vi "Fit VI window to Largest Dec.vi"(4 "error in (no error)":errorcluster, 6 "border spacing (2 px)":i32=2, 7 "VI Ref (calling VI)":refnum<vi>) -> (0 "error out":errorcluster, 3 "dup VI Ref":refnum<vi>)   [LabVIEW 2019]
doc: "This utility will fit (resize and center) a VI (defined by the \"VI Ref\" input) about the largest decoration in that VI. It will add a border defined by border spacing in units of pixels. If there are no decorations found in the VI it is a no-op and will not produce an error. Unfortunately, this VI can not find locked decorations (yet)."
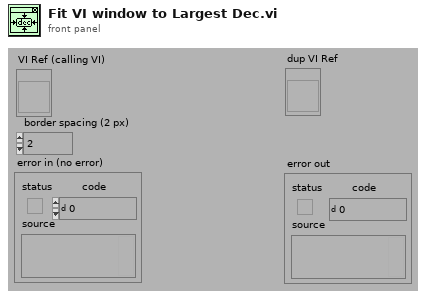
[diagram p1: front panel]
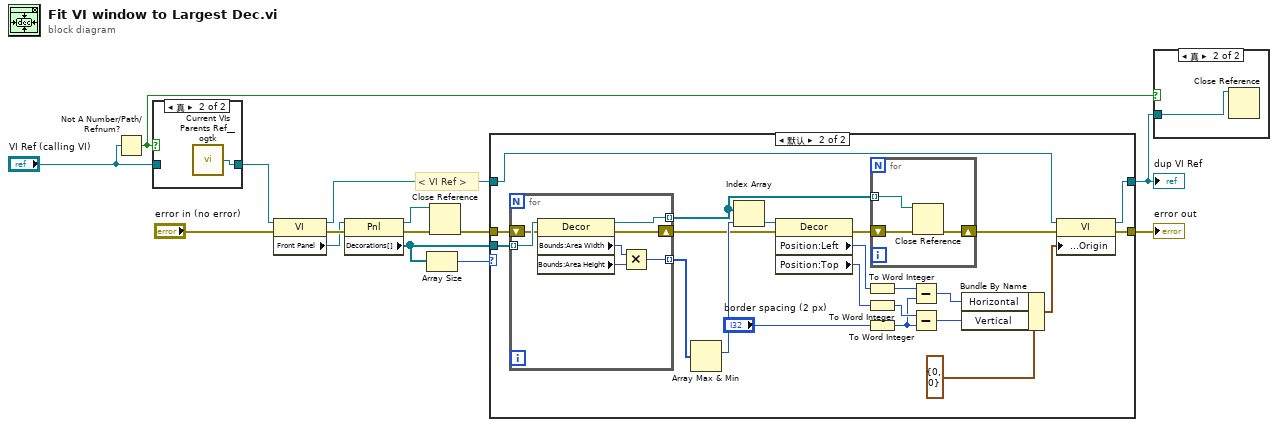
[diagram p0: block diagram]
diagram:
  # "< VI Ref >"
  n1 = Not A Number/Path/Refnum?(number/path/refnum="VI Ref (calling VI)") -> (NaN/Path/Refnum?=w2:bool)
  n2 = case shown="真" w2 {
    tunnel: [w15 w16] -> w3
    tunnel: "VI Ref (calling VI)" -> [w15 _]
    frame False {
    }
    frame True {
      n3 = call <userlib>:"Current VIs Parents Ref__ogtk.vi"() -> ("Calling VI's Reference"=w16:refnum<vi>)  [unwired: 2 in]
    }
  }
  n4 = property on="Property Node" class="VI"(reference=w3, error in="error in (no error)") -> (reference out=w14:refnum<vi>, error out=w12:errorcluster, "Front Panel"=w9:refnum<vi>)
  n5 = property on="Property Node" class="Pnl"(reference=w9, error in=w12) -> (reference out=w13:refnum<vi>, error out=w11:errorcluster, "Decorations[]"=w6:refnum<vi>[])
  n6 = Array Size(array=w6) -> (size(s)=w5:i32)
  n7 = Close Reference(reference=w13, error in (no error)=w11) -> (error out=w8:errorcluster)
  n8 = case shown="默认" w5 {
    tunnel: w14 -> [w18 w40]
    tunnel: w8 -> [w17 w33]
    tunnel: [w17 w20] -> w7
    tunnel: [w18 w19] -> w1
    tunnel: w6 -> [_ w24]
    frame 0 {
      # "do nothing if no decorations"
    }
    frame Default {
      n9 = for {
        tunnel: w24 -> [w47] mode=indexing
        tunnel: [w44] -> w32 mode=indexing
        shift-right: [w42] -> w28
        shift-left: w33 -> [w43]
        tunnel: [w41] -> w30 mode=indexing
        n10 = property class="Decor"(reference=w47, error in=w43) -> (reference out=w41:refnum<vi>, error out=w42:errorcluster, "Bounds:Area Width"=w46:u32, "Bounds:Area Height"=w45:u32)
        n11 = Multiply(x=w46, y=w45) -> (x*y=w44:u32)
      }
      n12 = Array Max & Min(array=w32) -> (max index (indices)=w31:i32)  [unwired: 3 out]
      n13 = Index Array(array=w30, index=w31) -> (element=w29:refnum<vi>)
      n14 = property class="Decor"(reference=w29, error in=w28) -> (error out=w27:errorcluster, "Position:Left"=w36:i32, "Position:Top"=w39:i32)  [unwired: 1 out]
      n15 = To Word Integer(number=w36) -> (16bit integer=w23:i16)
      n16 = To Word Integer(number=w39) -> (16bit integer=w22:i16)
      n17 = To Word Integer(number="border spacing (2 px)") -> (16bit integer=w21:i16)
      n18 = for {
        tunnel: w30 -> [w50] mode=indexing
        shift-right: [w48] -> w25
        shift-left: w27 -> [w49]
        n19 = Close Reference(reference=w50, error in (no error)=w49) -> (error out=w48:errorcluster)
      }
      n20 = Subtract(x=w23, y=w21) -> (x-y=w37:i16)
      n21 = Subtract(x=w22, y=w21) -> (x-y=w38:i16)
      n22 = Bundle By Name(cluster=cluster{"Horizontal":i16, "Vertical":i16} {"Horizontal"=0, "Vertical"=0} ("Front Panel Window:Origin"), "Horizontal"=w37, "Vertical"=w38) -> (w34:cluster{"Horizontal":i16, "Vertical":i16})
      n23 = property on="Property Node" class="VI"(reference=w40, error in=w25, "Front Panel Window:Origin"=w34) -> (reference out=w19:refnum<vi>, error out=w20:errorcluster)
    }
  }
  "error out" <- w7
  "dup VI Ref" <- w1
  n24 = case shown="真" w2 {
    tunnel: w1 -> [_ w51]
    frame False {
    }
    frame True {
      n25 = Close Reference(reference=w51) -> ()  [unwired: 1 in, 1 out]
    }
  }
